vi "w zakresie mapy.vi"(7 "Rozmiar mapy":T1={"left"=0, "top"=0, "right"=836, "bottom"=597}, 10 "Pixel x":i16, 11 "Pixel y":i16) -> (3 "Boolean":bool)   [LabVIEW 2015, in "Biblioteka moduł map v3.lvlib" / "Obsługa grafiki mapy.lvlib"]
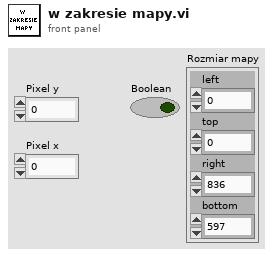
[diagram p1: front panel]
types:
  T1 = cluster{"left":i16, "top":i16, "right":i16, "bottom":i16}
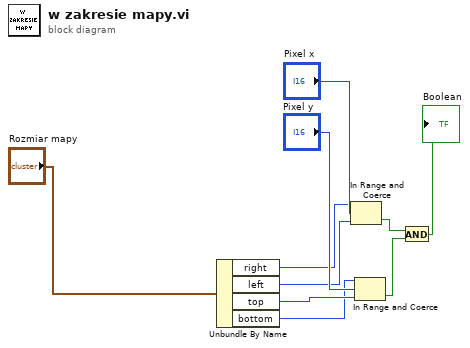
[diagram p0: block diagram]
diagram:
  n1 = Unbundle By Name("Rozmiar mapy") -> ("right"=w5:i16, "left"=w4:i16, "top"=w8:i16, "bottom"=w6:i16)
  n2 = In Range and Coerce(upper limit=w5, x="Pixel x", lower limit=w4) -> (In Range?=w2:bool)  [unwired: 1 out]
  n3 = In Range and Coerce(upper limit=w6, x="Pixel y", lower limit=w8) -> (In Range?=w3:bool)  [unwired: 1 out]
  n4 = And(x=w2, y=w3) -> (x .and. y?=→"Boolean":bool)
